vi "InitBallHandling.vi"   [LabVIEW 2019]
doc: "This VI initializes devices related directly to the intake, hopper, and magazine subsystems."
uses:
  <vilib>/Rock Robotics/WPI/Solenoid/WPI_SolenoidChannel.ctl
  <vilib>/Rock Robotics/WPI/ThirdParty/Phoenix-LabVIEW/Motor Controller/Controls/CTRE_Phoenix_MotorControl_SupplyCurrentLimitConfiguration.ctl
  <vilib>/Rock Robotics/WPI/ThirdParty/Phoenix-LabVIEW/Motor Controller/Controls/CTRE_Phoenix_MotorControl_TalonFXInvertType.ctl
  <vilib>/Rock Robotics/WPI/ThirdParty/Phoenix-LabVIEW/Motor Controller/Controls/CTRE_Phoenix_MotorControl_NeutralMode.ctl
  <vilib>/Rock Robotics/WPI/ThirdParty/Phoenix-LabVIEW/Motor Controller/Controls/CTRE_Phoenix_MotorControl_FeedbackDevice_TalonFX.ctl
  <vilib>/Rock Robotics/WPI/Solenoid/WPI_SolenoidOpenDouble.vi
  refnums.vi
types:
  T1 = typedef "CTRE_Phoenix_MotorControl_NeutralMode.ctl" = enum8{"EEPROMSetting", "Override to Coast", "Override to Brake"}
  T2 = typedef "CTRE_Phoenix_MotorControl_FeedbackDevice_TalonFX.ctl" = i8
  T3 = typedef "CTRE_Phoenix_MotorControl_TalonFXInvertType.ctl" = enum16{"Counter-Clockwise", "Clockwise"}
  T4 = typedef "CTRE_Phoenix_MotorControl_SupplyCurrentLimitConfiguration.ctl" = cluster{"Enable?":bool, "Current Limit":dbl, "Threshold Current":dbl, "Threshold Time":dbl}
  T5 = typedef "WPI_SolenoidChannel.ctl" = enum8{"Solenoid 0", "Solenoid 1", "Solenoid 2", "Solenoid 3", "Solenoid 4", "Solenoid 5", "Solenoid 6", "Solenoid 7", "Invalid"}
  T6 = typedef "WPI_MotorControlDeviceRef.ctl" = cluster{"DeviceStatus":errorcluster, "Type":T7, "PWM":cluster{"PWM Channel":T8, "DeadBand":T9}, "CAN":cluster{"Device Number":u8, "SetOutput VI Ref":variant, "GetOutput VI Ref":variant, "Enable VI Ref":variant, "Disable VI Ref":variant, "Data":variant}, "Invert":bool, "DIO PWM":cluster{"PWM \"Enable\" Channel":T8, "DIOChannel":T10, "PWM Rate":dbl}}
  T7 = typedef "WPI_MotorControlType.ctl" = enum16{"PWM", "CAN", "DIO PWM"}
  T8 = typedef "FPGA_DIOPWMChannel.ctl" = enum8{"PWM 0", "PWM 1", "PWM 2", "PWM 3", "PWM 4", "PWM 5", "PWM 6", "PWM 7", "PWM 8", "PWM 9", "PWM MXP 0", "PWM MXP 1", "PWM MXP 2", "PWM MXP 3", "PWM MXP 4", "PWM MXP 5", "PWM MXP 6", "PWM MXP 7", "PWM MXP 8", "PWM MXP 9", "Invalid"}
  T9 = typedef "WPI_PWMDeadband.ctl" = cluster{"Name":string, "maxPositivePwm":i32, "minPositivePwm":i32, "centerPwm":i32, "maxNegativePwm":i32, "minNegativePwm":i32, "angularRange":u16}
  T10 = typedef "FPGA_DIOChannel.ctl" = enum8{"DIO 0", "DIO 1", "DIO 2", "DIO 3", "DIO 4", "DIO 5", "DIO 6", "DIO 7", "DIO 8", "DIO 9", "DIO MXP 0", "DIO MXP 1", "DIO MXP 2", "DIO MXP 3", "DIO MXP 4", "DIO MXP 5", "DIO MXP 6", "DIO MXP 7", "DIO MXP 8", "DIO MXP 9", "DIO MXP 10", "DIO MXP 11", "DIO MXP 12", "DIO MXP 13", "DIO MXP 14", "DIO MXP 15", "SPI Port CS1", "SPI Port CS2", "SPI Port CS3", "SPI Port MISO", "SPI Port MOSI", "Invalid"}
  T11 = typedef "WPI_SolenoidDevRef.ctl" = cluster{"DevStatus":errorcluster, "Pneumatics Control Module":u8, "Forward Solenoid Channel":T5, "Reverse Solenoid Channel":T5}
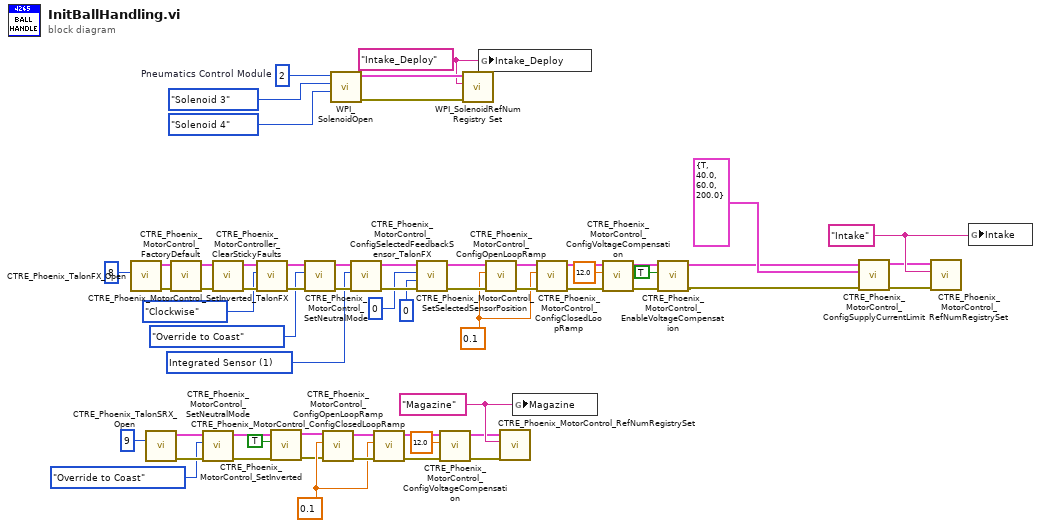
[diagram p0: block diagram]
diagram:
  w6 = 0.1 ("secondsFromNeutralToFull")
  w11 = "Magazine" ("refnum name")
  w21 = 0.1 ("secondsFromNeutralToFull")
  w23 = T2 1 items=["Integrated Sensor"=1, "Sensor Sum (S0 + S1)"=9, "Sensor Difference (D0 - D1)"=10, "Remote Source 0"=11, "Remote Source 1"=12, "None"=14, "Software Emulated"=15] ("Talon FX Feedback Device")
  w49 = "Intake" ("refnum name")
  w54 = "Intake_Deploy" ("refnum name")
  w59 = u8 2  # Pneumatics Control Module
  n1 = call <vilib>:"CTRE_Phoenix_TalonFX_Open.vi"("Device Number"=u8 8 ("Drive 4L")) -> ("error out"=w38:errorcluster, "CAN Talon SRX Ref"=w45:T6)  [unwired: 9 in]
  n2 = call <vilib>:"CTRE_Phoenix_TalonSRX_Open.vi"("Device Number"=u8 9) -> ("error out"=w18:errorcluster, "CAN Talon SRX Ref"=w17:T6)  [unwired: 9 in]
  n3 = call <vilib>:"CTRE_Phoenix_MotorControl_FactoryDefault.vi"("error in"=w38, "PhoenixMotorControlDevRef"=w45) -> ("error out"=w41:errorcluster, "PhoenixMotorControlDevRef"=w42:T6)  [unwired: 8 in]
  n4 = call <vilib>:"CTRE_Phoenix_MotorControl_SetNeutralMode.vi"("error in (no error)"=w18, "Motor Control Neutral Mode"=CTRE_Phoenix_MotorControl_NeutralMode."Override to Coast", "PhoenixMotorControlDevRef"=w17) -> ("error out"=w16:errorcluster, "PhoenixMotorControlDevRef"=w15:T6)  [unwired: 7 in]
  n5 = call <vilib>:"CTRE_Phoenix_MotorController_ClearStickyFaults.vi"("error in"=w41, "PhoenixMotorControlDevRef"=w42) -> ("error out"=w40:errorcluster, "PhoenixMotorControlDevRef"=w39:T6)  [unwired: 8 in]
  n6 = call <vilib>:"CTRE_Phoenix_MotorControl_SetInverted_TalonFX.vi"("error in (no error)"=w40, "Invert Type"=CTRE_Phoenix_MotorControl_TalonFXInvertType."Clockwise", "PhoenixMotorControlDevRef"=w39) -> ("error out"=w52:errorcluster, "PhoenixMotorControlDevRef"=w53:T6)  [unwired: 7 in]
  n7 = call <vilib>:"CTRE_Phoenix_MotorControl_SetInverted.vi"("error in (no error)"=w16, "Invert?"=TRUE, "PhoenixMotorControlDevRef"=w15) -> ("error out"=w3:errorcluster, "PhoenixMotorControlDevRef"=w4:T6)  [unwired: 7 in]
  n8 = call <vilib>:"CTRE_Phoenix_MotorControl_SetNeutralMode.vi"("error in (no error)"=w52, "Motor Control Neutral Mode"=CTRE_Phoenix_MotorControl_NeutralMode."Override to Coast", "PhoenixMotorControlDevRef"=w53) -> ("error out"=w36:errorcluster, "PhoenixMotorControlDevRef"=w37:T6)  [unwired: 7 in]
  n9 = call <vilib>:"CTRE_Phoenix_MotorControl_ConfigOpenLoopRamp.vi"("error in (no error)"=w3, "secondsFromNeutralToFull"=w6, "PhoenixMotorControlDevRef"=w4) -> ("error out"=w9:errorcluster, "PhoenixMotorControlDevRef"=w10:T6)  [unwired: 7 in]
  n10 = call-poly <vilib>:"WPI_SolenoidOpen.vi"("Reverse Solenoid Channel"=WPI_SolenoidChannel."Solenoid 4", "Forward Solenoid Channel"=WPI_SolenoidChannel."Solenoid 3", "Pneumatics Control Module (0)"=w59) -> ("error out"=w55:errorcluster, "SolenoidDevRef"=w56:T11)  [unwired: 7 in]
  n11 = call <vilib>:"CTRE_Phoenix_MotorControl_ConfigSelectedFeedbackSensor_TalonFX.vi"("error in (no error)"=w36, "Talon FX Feedback Device"=w23, "PhoenixMotorControlDevRef"=w37) -> ("error out"=w34:errorcluster, "PhoenixMotorControlDevRef"=w35:T6)  [unwired: 7 in]
  n12 = call <vilib>:"CTRE_Phoenix_MotorControl_ConfigClosedLoopRamp.vi"("error in (no error)"=w9, "secondsFromNeutralToFull"=w6, "PhoenixMotorControlDevRef"=w10) -> ("error out"=w7:errorcluster, "PhoenixMotorControlDevRef"=w8:T6)  [unwired: 7 in]
  n13 = call <vilib>:"CTRE_Phoenix_MotorControl_SetSelectedSensorPosition.vi"("error in (no error)"=w34, "pidLoopIdx"=u32 0, "New Sensor Position"=0, "PhoenixMotorControlDevRef"=w35) -> ("error out"=w51:errorcluster, "PhoenixMotorControlDevRef"=w50:T6)  [unwired: 6 in]
  n14 = call <vilib>:"CTRE_Phoenix_MotorControl_ConfigVoltageCompensation.vi"("error in (no error)"=w7, "Saturation Voltage"=12.0, "PhoenixMotorControlDevRef"=w8) -> ("error out"=w1:errorcluster, "PhoenixMotorControlDevRef"=w2:T6)  [unwired: 7 in]
  n15 = call <vilib>:"WPI_SolenoidRefNum Registry Set.vi"("error in (no error)"=w55, "refnum name"=w54, "SolenoidDevRef"=w56) -> ()  [unwired: 7 in, 2 out]
  n16 = global write "refnums.vi" "Intake_Deploy"(w54) -> ()
  n17 = call <vilib>:"CTRE_Phoenix_MotorControl_ConfigOpenLoopRamp.vi"("error in (no error)"=w51, "secondsFromNeutralToFull"=w21, "PhoenixMotorControlDevRef"=w50) -> ("error out"=w43:errorcluster, "PhoenixMotorControlDevRef"=w44:T6)  [unwired: 7 in]
  n18 = call <vilib>:"CTRE_Phoenix_MotorControl_RefNumRegistrySet.vi"("error in (no error)"=w1, "refnum name"=w11, "PhoenixMotorControlDevRef"=w2) -> ()  [unwired: 7 in, 2 out]
  n19 = global write "refnums.vi" "Magazine"(w11) -> ()
  n20 = call <vilib>:"CTRE_Phoenix_MotorControl_ConfigClosedLoopRamp.vi"("error in (no error)"=w43, "secondsFromNeutralToFull"=w21, "PhoenixMotorControlDevRef"=w44) -> ("error out"=w28:errorcluster, "PhoenixMotorControlDevRef"=w29:T6)  [unwired: 7 in]
  n21 = call <vilib>:"CTRE_Phoenix_MotorControl_ConfigVoltageCompensation.vi"("error in (no error)"=w28, "Saturation Voltage"=12.0, "PhoenixMotorControlDevRef"=w29) -> ("error out"=w30:errorcluster, "PhoenixMotorControlDevRef"=w31:T6)  [unwired: 7 in]
  n22 = call <vilib>:"CTRE_Phoenix_MotorControl_EnableVoltageCompensation.vi"("error in (no error)"=w30, "Enable Voltage Compensation?"=TRUE, "PhoenixMotorControlDevRef"=w31) -> ("error out"=w26:errorcluster, "PhoenixMotorControlDevRef"=w27:T6)  [unwired: 7 in]
  n23 = call <vilib>:"CTRE_Phoenix_MotorControl_ConfigSupplyCurrentLimit.vi"("error in (no error)"=w26, "Supply Current Limit Configuration"=T4 {"Enable?"=TRUE, "Current Limit"=40.0, "Threshold Current"=60.0, "Threshold Time"=200.0}, "PhoenixMotorControlDevRef"=w27) -> ("error out"=w47:errorcluster, "PhoenixMotorControlDevRef"=w48:T6)  [unwired: 7 in]
  n24 = call <vilib>:"CTRE_Phoenix_MotorControl_RefNumRegistrySet.vi"("error in (no error)"=w47, "refnum name"=w49, "PhoenixMotorControlDevRef"=w48) -> ()  [unwired: 7 in, 2 out]
  n25 = global write "refnums.vi" "Intake"(w49) -> ()
